vi "Parse for Instrument Name.vi"(9 "Instrument Name":string, 10 "Message In":T1, 11 "Message Queue":refnum<queue>) -> (3 "Message Out":T1)   [LabVIEW 2014, in "MeasurementControl Message Queue.lvlib"]
doc: "This VI determine if a message to the master queue is sent to the correct instrument. If so, it is passed through the the instrument's UI queue. If not, it is ignored."
uses:
  MeasurementControl Message Queue.lvlib
  Message Cluster.ctl
  <vilib>/regexp/Match Regular Expression.xnode
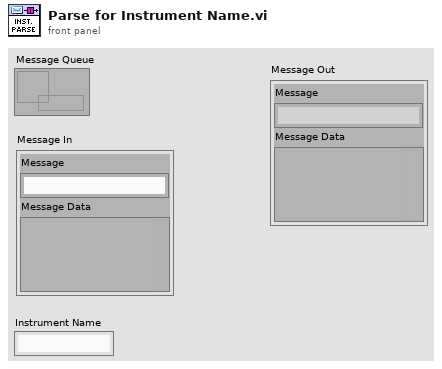
[diagram p1: front panel]
types:
  T1 = typedef "MeasurementControl Message Queue.lvlib/Message Cluster.ctl" = cluster{"Message":string, "Message Data":variant}
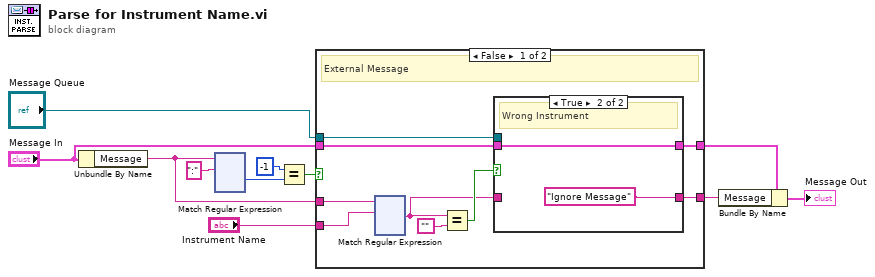
[diagram p0: block diagram]
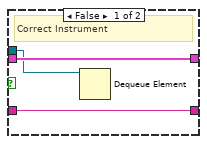
[diagram p2: hidden frame]
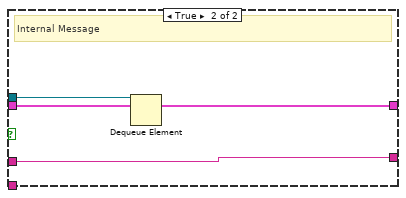
[diagram p3: hidden frame]
diagram:
  n1 = Unbundle By Name("Message In") -> ("Message"=w6:string)
  n2 = xnode "Match Regular Expression"("input string"=w6, "regular expression"=":") -> ("offset past match"=w10:i32)  [unwired: 4 in, 4 out]
  n3 = Equal?(x=-1, y=w10) -> (x = y?=w8:bool)
  n4 = case shown="False" w8 {
    tunnel: [w15 w142] -> w3
    tunnel: "Instrument Name" -> [w20 _]
    tunnel: w6 -> [w18 w142]
    tunnel: "Message Queue" -> [w14 w140]
    tunnel: "Message In" -> [w13 w141]
    tunnel: [w12 w141] -> w1
    frame False {
      # "External Message"
      n5 = xnode "Match Regular Expression"("input string"=w18, "regular expression"=w20) -> ("after match"=w16:string)  [unwired: 4 in, 4 out]
      n6 = Equal?(x=w16, y="") -> (x = y?=w17:bool)
      n7 = case shown="True" w17 {
        tunnel: w16 -> [w23 _]
        tunnel: [w23 "Ignore Message" ("t")] -> w15
        tunnel: w14 -> [w21 _]
        tunnel: w13 -> [w22 w24]
        tunnel: [w22 w24] -> w12
        frame False {
          # "Correct Instrument"
          n8 = Dequeue Element(queue=w21) -> ()  [unwired: 2 in, 4 out]
        }
        frame True {
          # "Wrong Instrument"
        }
      }
    }
    frame True {
      # "Internal Message"
      n9 = Dequeue Element(queue=w140) -> ()  [unwired: 2 in, 4 out]
    }
  }
  n10 = Bundle By Name(cluster=w1, "Message"=w3) -> (→"Message Out":T1)
